vi "4Pi 4Pi Modes - Select Modes.vi"() -> ()   [LabVIEW 2016]
uses:
  4Pi 4Pi Modes - Controls/4Pi 4Pi Modes - Mirror Modes.ctl
  <vilib>/Utility/miscctls.llb/LVPointTypeDef.ctl
  Hardware Configuration/Hardware Configuration Controls/Standard Action.ctl
  4Pi 4Pi Modes - Controls/4Pi 4Pi Modes - Standard Action.ctl
  <userlib>/BMC/BMC.lvlib
panel:
  in  "DM index":string(combo)="0"
  in  "Mirror Modes":T1
  in  "Flags":string="--help"
  in  "Run":bool
  out "error":errorcluster
  out "standard output":string
  out "standard error":string
  in  "Control mode":string(combo)="Single"
  in  "Calling VI Ref":refnum<vi>
  in  "Help":bool
  in  "Quit":bool
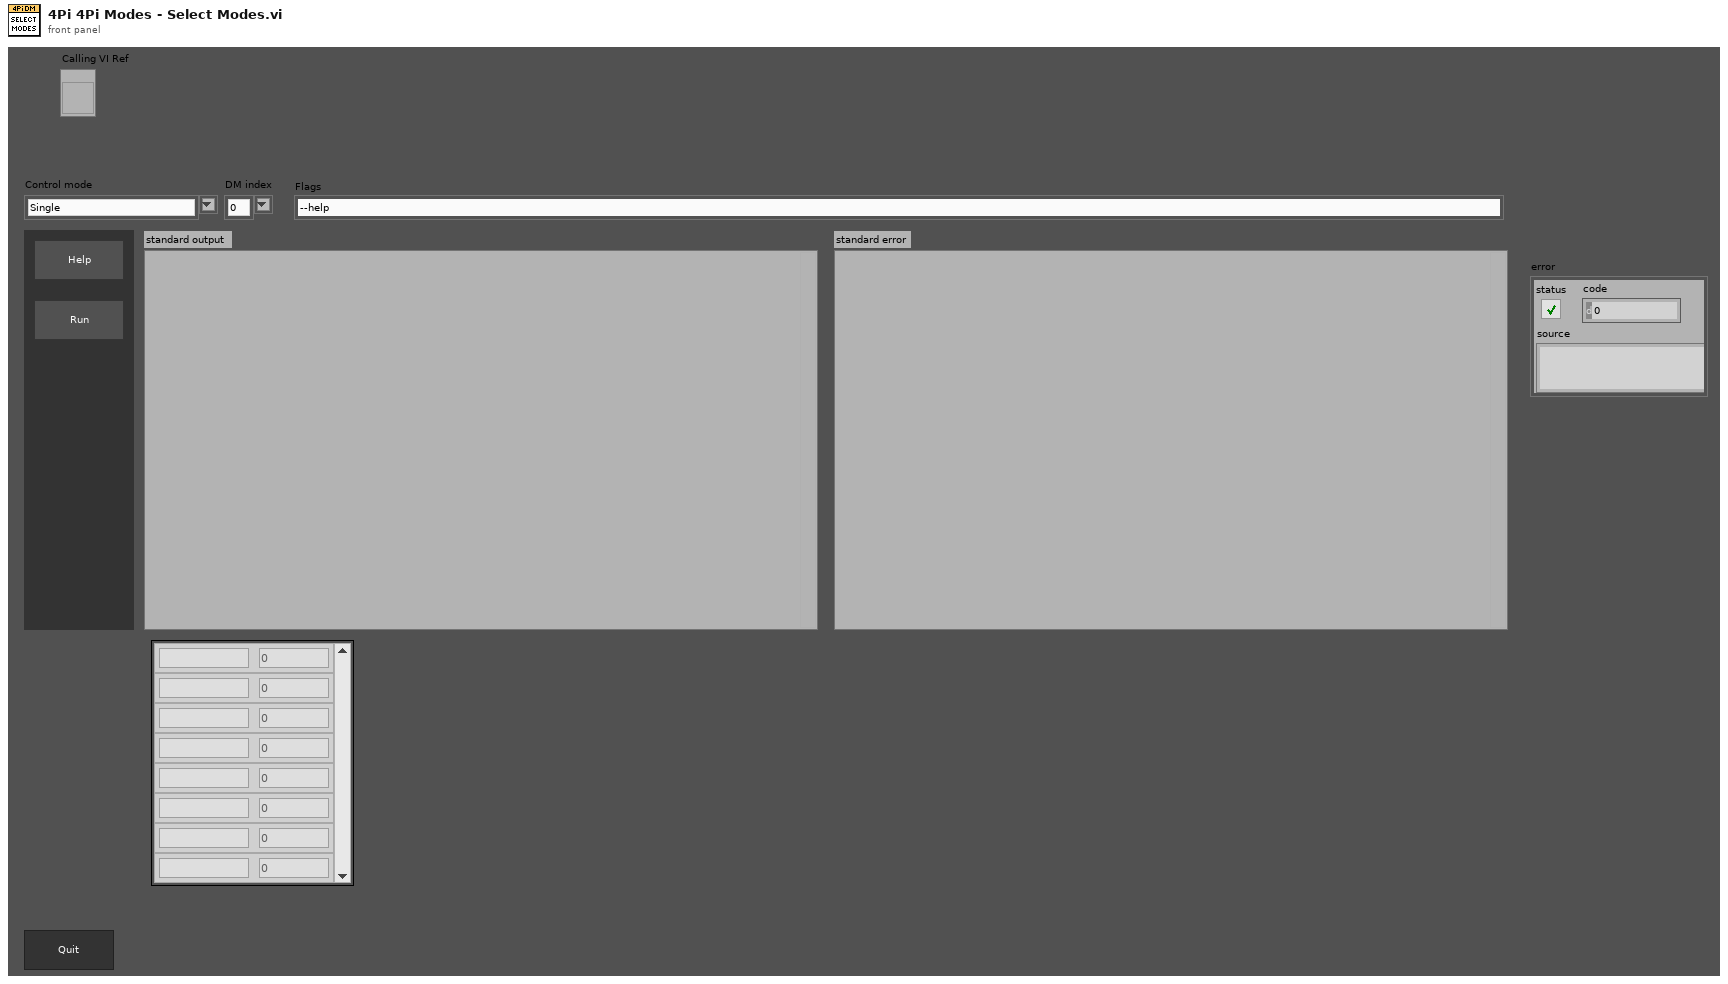
[diagram p1: front panel]
types:
  T1 = typedef "4Pi 4Pi Modes - Mirror Modes.ctl" = cluster{"Mode":string, "Amplitude":dbl}[]
  T2 = enum16{"Always On", "Always Off", "Off While Running"}
  T3 = typedef "LVPointTypeDef.ctl" = cluster{"Horizontal":i16, "Vertical":i16}
  T4 = typedef "Standard Action.ctl" = enum16{"Read", "Write"}
  T5 = typedef "4Pi 4Pi Modes - Standard Action.ctl" = enum16{"Read", "Write"}
  T6 = cluster{"type":i16, "ID":i16, "size":i32, "lutName":u64, "priv":u64}[]
  T7 = typedef "LVRectTypeDef.ctl" = cluster{"Left":i16, "Top":i16, "Right":i16, "Bottom":i16}
  T8 = typedef "LVBoundsTypeDef.ctl" = cluster{"Width":u32, "Height":u32}
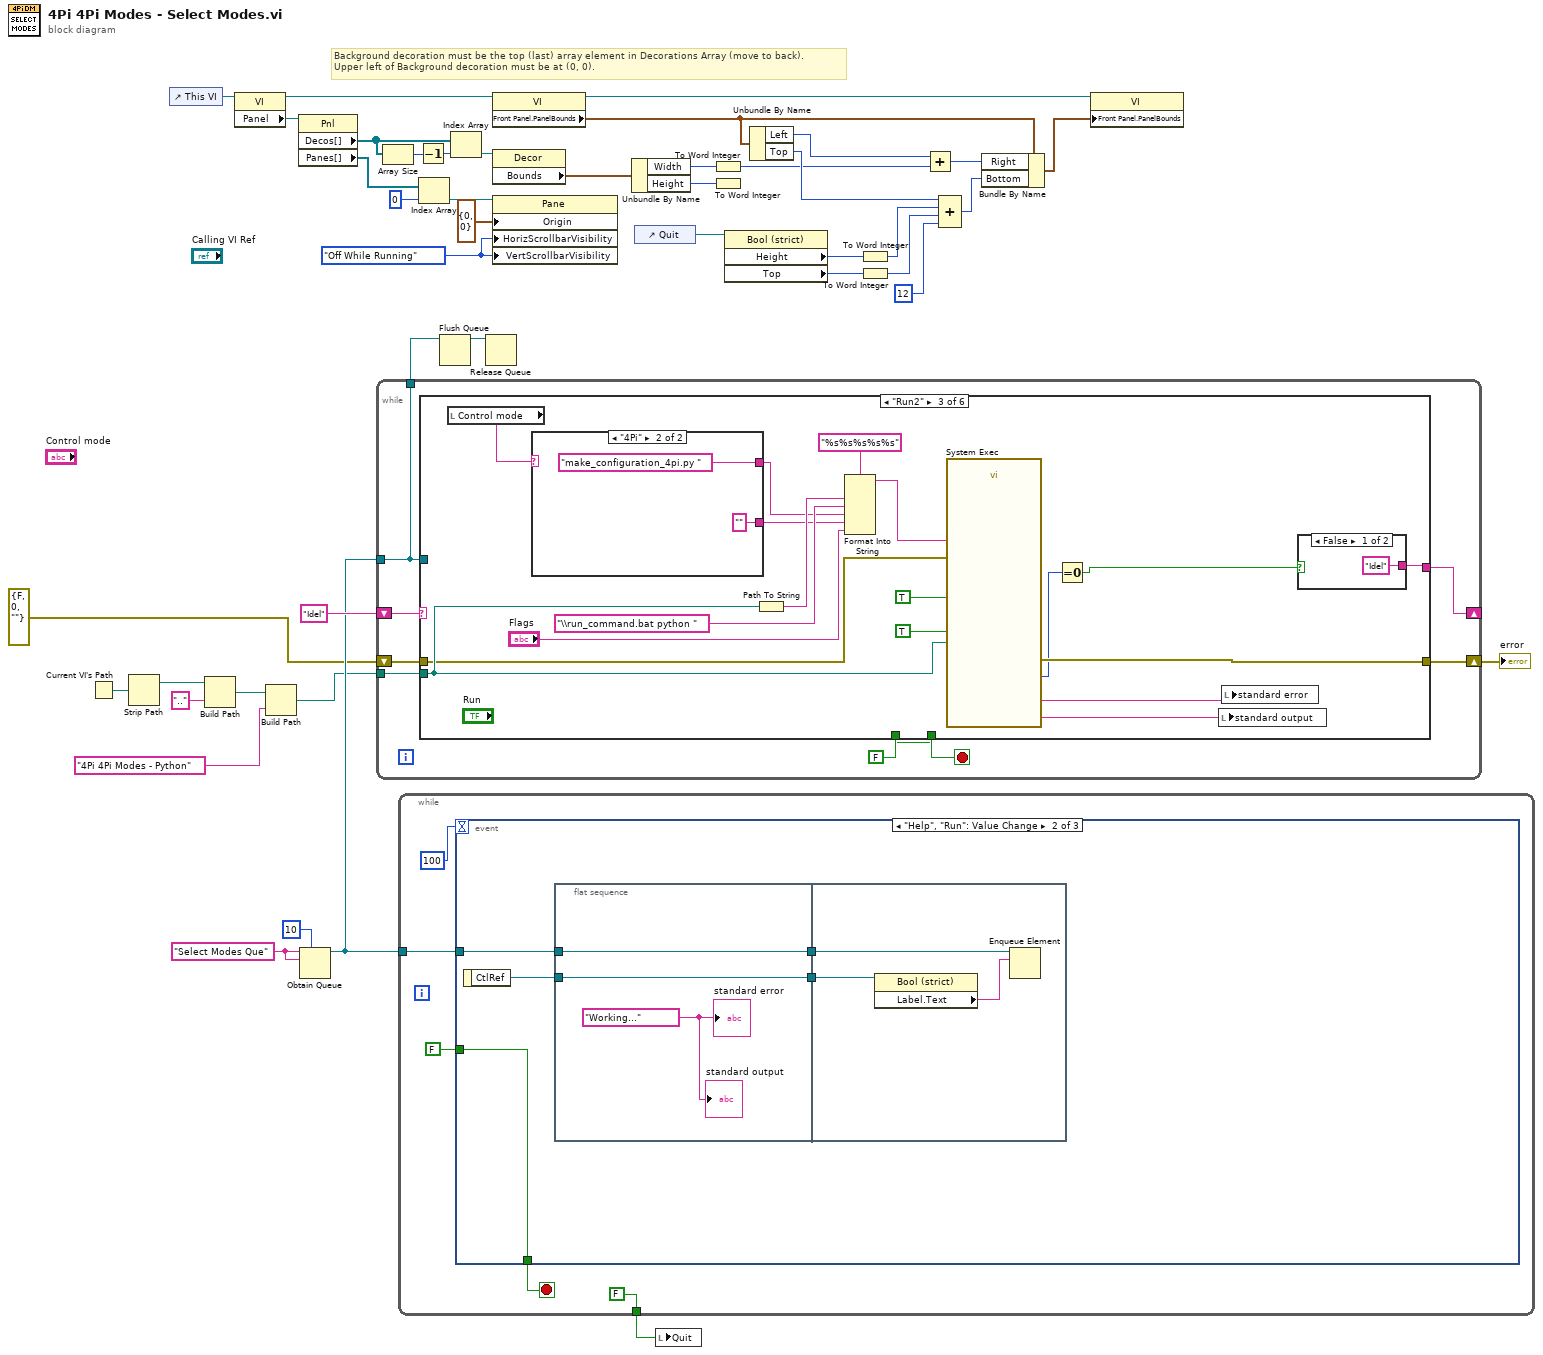
[diagram p0: block diagram]
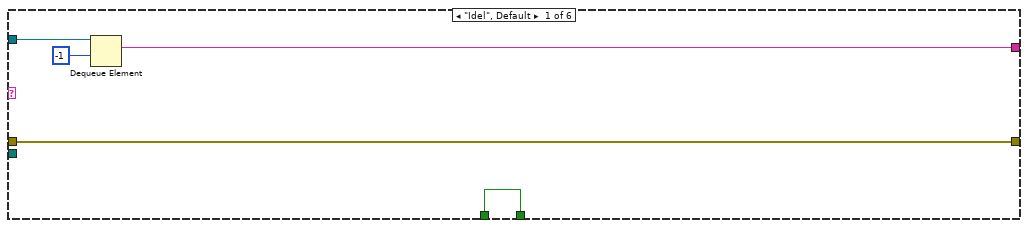
[diagram p2: hidden frame]
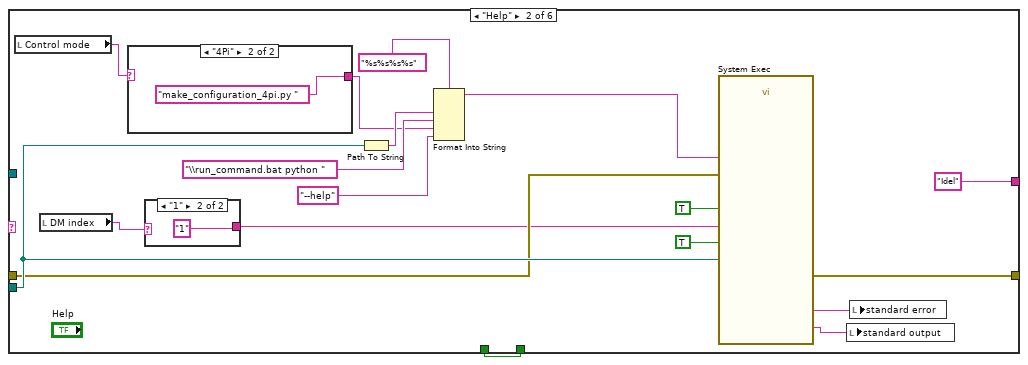
[diagram p3: hidden frame]
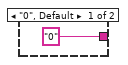
[diagram p4: hidden frame]
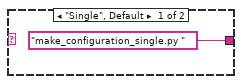
[diagram p5: hidden frame]
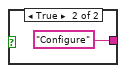
[diagram p6: hidden frame]
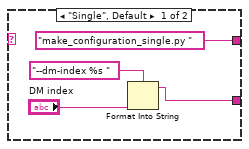
[diagram p7: hidden frame]
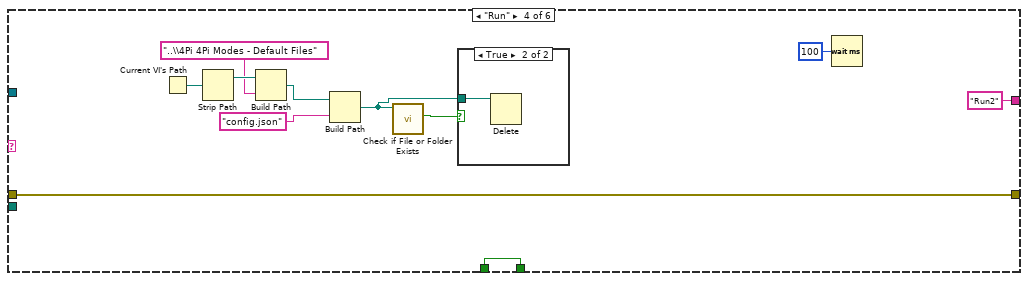
[diagram p8: hidden frame]
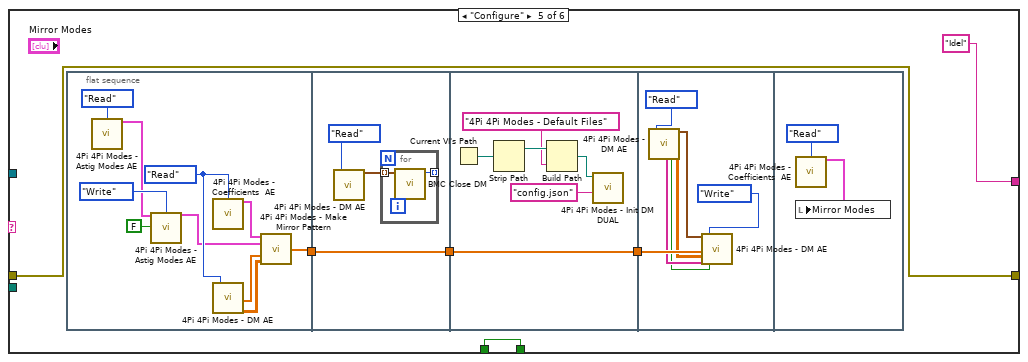
[diagram p10: hidden frame]
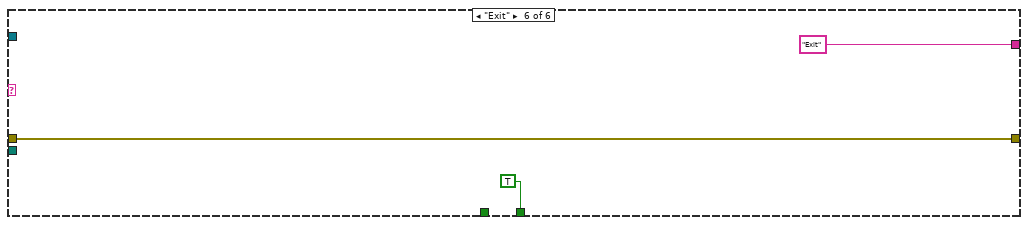
[diagram p11: hidden frame]
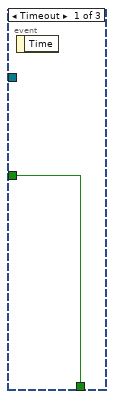
[diagram p12: hidden frame]
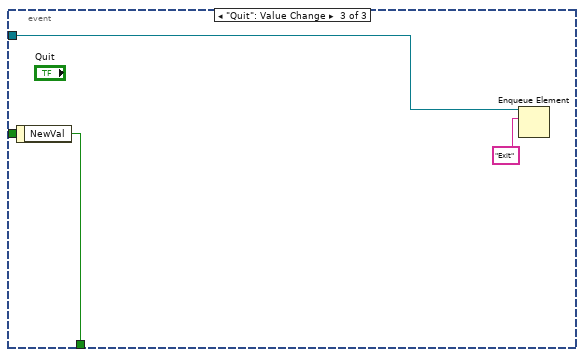
[diagram p13: hidden frame]
diagram:
  w21 = T2."Off While Running" ("Vertical Scrollbar Visibility")
  w44 = "Select Modes Que" ("name (unnamed)")
  # "Background decoration must be the top (last) array element in Decorations Array (move to back).\nUpper left of Background decoration must be at (0, 0)."
  n1 = Current VI's Path() -> (path=w7:path)
  n2 = Strip Path(path=w7) -> (stripped path=w6:path)  [unwired: 1 out]
  n3 = control-ref of="This VI"() -> (w13:refnum<vi>)
  n4 = Build Path(base path=w6, name or relative path="..") -> (appended path=w3:path)
  n5 = property class="VI"(reference=w13) -> (reference out=w22:refnum<vi>, "Panel"=w14:refnum<vi>)  [unwired: 1 in, 1 out]
  n6 = Build Path(base path=w3, name or relative path="4Pi 4Pi Modes - Python") -> (appended path=w4:path)
  n7 = property class="Pnl"(reference=w14) -> ("Decos[]"=w12:refnum<vi>[], "Panes[]"=w18:refnum<vi>[])  [unwired: 1 in, 2 out]
  n8 = Obtain Queue(max queue size (-1, unlimited)=10, name (unnamed)=w44, element data type=w44) -> (queue out=w39:refnum<queue>)  [unwired: 2 in, 2 out]
  n9 = while {
    tunnel: w39 -> [w48]
    shift-right: [w52] -> _
    shift-left: "Idel" ("name (unnamed)") -> [w51]
    tunnel: [w48] -> w42
    tunnel: w4 -> [w47]
    shift-right: [w46] -> w2
    shift-left: errorcluster {"status"=FALSE, "code"=0, "source"=""} ("error out") -> [w45]
    stop <- w50 stop-if-true
    n10 = case shown="\"Run2\"" w51 {
      tunnel: w48 -> [w57 _ _ _ _ _]
      tunnel: [w55 "Idel" ("name (unnamed)") w82 "Run2" ("name (unnamed)") "Idel" ("name (unnamed)") "Exit" ("name (unnamed)")] -> w52
      tunnel: [w54 w74 w98 w110 w119 TRUE] -> w50
      tunnel: FALSE -> [w54 w74 w98 w110 w119 _]
      tunnel: w47 -> [_ w67 w91 _ _ _]
      tunnel: [w53 w60 w86 w111 w120 w155] -> w46
      tunnel: w45 -> [w53 w61 w85 w111 w120 w155]
      frame "Idel", Default {
        n11 = Dequeue Element(queue=w57, timeout in ms (-1)=-1) -> (element=w55:string)  [unwired: 1 in, 3 out]
      }
      frame "Help" {
        n12 = local read "Control mode"() -> (w69:string)
        n13 = local read "DM index"() -> (w59:string)
        n14 = case shown="\"4Pi\"" w69 {
          tunnel: ["make_configuration_single.py " "make_configuration_4pi.py "] -> w63
          frame "Single", Default {
          }
          frame "4Pi" {
          }
        }
        n15 = case shown="\"1\"" w59 {
          tunnel: ["0" ("name or relative path") "1" ("name or relative path")] -> w58
          frame "0", Default {
          }
          frame "1" {
          }
        }
        n16 = Path To String(path=w67) -> (string=w66:string)
        n17 = Format Into String(format string="%s%s%s%s", w66, "\\run_command.bat python " ("name or relative path"), w63, "--help" ("name or relative path")) -> (resulting string=w64:string)  [unwired: 2 in, 1 out]
        n18 = call <vilib>:"System Exec.vi"("run minimized? (F)"=TRUE, "wait until completion? (T)"=TRUE, "error in (no error)"=w61, "working directory"=w67, "standard input"=w58, "command line"=w64) -> ("error out"=w60:errorcluster, "standard error"=w71:string, "standard output"=w70:string)  [unwired: 2 in, 1 out]
        n19 = local write "standard output"(w70) -> ()
        n20 = local write "standard error"(w71) -> ()
      }
      frame "Run2" {
        n21 = local read "Control mode"() -> (w93:string)
        n22 = case shown="\"4Pi\"" w93 {
          tunnel: ["make_configuration_single.py " "make_configuration_4pi.py "] -> w87
          tunnel: [w101 ""] -> w80
          frame "Single", Default {
            n23 = Format Into String(format string="--dm-index %s ", "DM index") -> (resulting string=w101:string)  [unwired: 2 in, 1 out]
          }
          frame "4Pi" {
          }
        }
        n24 = Path To String(path=w91) -> (string=w90:string)
        n25 = Format Into String(format string="%s%s%s%s%s", w90, "\\run_command.bat python " ("name or relative path"), w87, w80, "Flags") -> (resulting string=w88:string)  [unwired: 2 in, 1 out]
        n26 = call <vilib>:"System Exec.vi"("run minimized? (F)"=TRUE, "wait until completion? (T)"=TRUE, "error in (no error)"=w85, "working directory"=w91, "command line"=w88) -> ("error out"=w86:errorcluster, "return code"=w84:i32, "standard error"=w95:string, "standard output"=w94:string)  [unwired: 3 in]
        n27 = Equal To 0?(x=w84) -> (x = 0?=w83:bool)
        n28 = local write "standard output"(w94) -> ()
        n29 = local write "standard error"(w95) -> ()
        n30 = case shown="False" w83 {
          tunnel: ["Idel" ("name (unnamed)") "Configure" ("name (unnamed)")] -> w82
          frame False {
          }
          frame True {
          }
        }
      }
      frame "Run" {
        n31 = Current VI's Path() -> (path=w116:path)
        n32 = Strip Path(path=w116) -> (stripped path=w117:path)  [unwired: 1 out]
        n33 = Build Path(base path=w117, name or relative path="..\\4Pi 4Pi Modes - Default Files") -> (appended path=w114:path)
        n34 = Build Path(base path=w114, name or relative path="config.json") -> (appended path=w107:path)
        n35 = call <vilib>:"Check if File or Folder Exists.vi"("path"=w107) -> ("file or folder exists?"=w108:bool)  [unwired: 8 in, 2 out]
        n36 = case shown="True" w108 {
          tunnel: w107 -> [_ w118]
          frame False {
          }
          frame True {
            n37 = Delete(path (use dialog)=w118) -> ()  [unwired: 4 in, 3 out]
          }
        }
        n38 = Wait (ms)(milliseconds to wait=u32 100) -> ()  [unwired: 1 out]
      }
      frame "Configure" {
        n39 = flat-sequence {
          tunnel: [w125] -> w124
          tunnel: w124 -> [w137]
          tunnel: [w137] -> w123
          tunnel: w123 -> [w140]
          tunnel: [w140] -> w122
          tunnel: w122 -> [w149]
          frame #0 {
            w131 = 4Pi_4Pi_Modes_-_Standard_Action."Read" ("Action")
            n40 = call "4Pi 4Pi Modes - Astig Modes AE.vi"("Action"=Standard_Action."Read") -> ("Coefficients Out"=w126:cluster{"Mode":string, "Amplitude":dbl}[])  [unwired: 13 in, 1 out]
            n41 = call "4Pi 4Pi Modes - Astig Modes AE.vi"("Coefficients In"=w126, "Action"=Standard_Action."Write", "Enabled In"=FALSE) -> ("Coefficients Out"=w129:cluster{"Mode":string, "Amplitude":dbl}[])  [unwired: 11 in, 1 out]
            n42 = call "4Pi 4Pi Modes - Coefficients  AE.vi"("Action"=w131) -> ("Coefficients Out"=w130:cluster{"Mode":string, "Amplitude":dbl}[])  [unwired: 14 in]
            n43 = call "4Pi 4Pi Modes - DM AE.vi"("Action"=w131) -> ("Flats Out"=w128:dbl[], "Control Matrix Out"=w127:dbl[][])  [unwired: 14 in, 3 out]
            n44 = call "4Pi 4Pi Modes - Make Mirror Pattern.vi"("Coefficients"=w130, "Astig Coeffs"=w129, "Flats"=w128, "Control Matrix"=w127) -> ("Pixel Value U (-1 to 1)"=w125:dbl[])  [unwired: 10 in, 1 out]
          }
          frame #1 {
            n45 = call "4Pi 4Pi Modes - DM AE.vi"("Action"=4Pi_4Pi_Modes_-_Standard_Action."Read") -> ("DM Handles Out"=w135:T6)  [unwired: 14 in, 4 out]
            n46 = for {
              tunnel: w135 -> [w139] mode=indexing
              tunnel: [w138] -> _ mode=indexing
              n47 = call <userlib>:"BMC Close DM.vi"("dmHandle"=w139) -> ("function return"=w138:i32)  [unwired: 9 in, 1 out]
            }
          }
          frame #2 {
            n48 = Current VI's Path() -> (path=w142:path)
            n49 = Strip Path(path=w142) -> (stripped path=w143:path)  [unwired: 1 out]
            n50 = Build Path(base path=w143, name or relative path="4Pi 4Pi Modes - Default Files") -> (appended path=w145:path)
            n51 = call "4Pi 4Pi Modes - Init DM DUAL.vi"("Config File"="config.json" ("name or relative path"), "Base File Path"=w145) -> ()  [unwired: 8 in, 2 out]
          }
          frame #3 {
            n52 = call "4Pi 4Pi Modes - DM AE.vi"("Action"=4Pi_4Pi_Modes_-_Standard_Action."Read") -> ("Serials Out"=w147:string[], "No hardware Out"=w146:bool, "DM Handles Out"=w150:T6, "Control Matrix Out"=w148:dbl[][])  [unwired: 14 in, 1 out]
            n53 = call "4Pi 4Pi Modes - DM AE.vi"("DM Handles"=w150, "Flats"=w149, "Control Matrix"=w148, "Serials"=w147, "Action"=4Pi_4Pi_Modes_-_Standard_Action."Write", "No hardware"=w146) -> ()  [unwired: 9 in, 5 out]
          }
          frame #4 {
            n54 = call "4Pi 4Pi Modes - Coefficients  AE.vi"("Action"=4Pi_4Pi_Modes_-_Standard_Action."Read") -> ("Coefficients Out"=w153:cluster{"Mode":string, "Amplitude":dbl}[])  [unwired: 14 in]
            n55 = local write "Mirror Modes"(w153) -> ()
          }
        }
      }
      frame "Exit" {
      }
    }
  }
  "error" <- w2
  n56 = Array Size(array=w12) -> (size(s)=w10:i32)
  n57 = while {
    tunnel: w39 -> [w159]
    tunnel: [FALSE] -> w9
    stop <- w162 stop-if-true
    n58 = event shown="[1] \"Help\", \"Run\": Value Change" {
      selector: _ -> [_ _ _]
      dyn-events: _ -> [_ _ _]
      timeout: 100 -> [_ _ _]
      tunnel: [w163 w168 w177] -> w162
      tunnel: FALSE -> [w163 w168 _]
      tunnel: w159 -> [_ w167 w175]
      event Timeout {
        n59 = event-data() -> ()  [unwired: 1 in, 1 out]
      }
      event "Help", "Run": Value Change {
        n60 = event-data() -> ("CtlRef"=w166:refnum<vi>)  [unwired: 1 in]
        n61 = flat-sequence {
          tunnel: w166 -> [w170]
          tunnel: w167 -> [w171]
          tunnel: [w171] -> w165
          tunnel: [w170] -> w164
          tunnel: w165 -> [w174]
          tunnel: w164 -> [w173]
          frame #0 {
            w169 = "Working..." ("standard error")
            "standard error" <- w169
            "standard output" <- w169
          }
          frame #1 {
            n62 = property class="Bool (strict)"(reference=w173) -> ("Label.Text"=w172:string)  [unwired: 1 in, 2 out]
            n63 = Enqueue Element(queue=w174, element=w172) -> ()  [unwired: 2 in, 3 out]
          }
        }
      }
      event "Quit": Value Change {
        n64 = event-data() -> ("NewVal"=w177:bool)  [unwired: 1 in]
        n65 = Enqueue Element(queue=w175, element="Exit") -> ()  [unwired: 2 in, 3 out]
      }
    }
  }
  n66 = Decrement(x=w10) -> (x-1=w11:i32)
  n67 = Index Array(array=w18, index=0) -> (element=w17:refnum<vi>)
  n68 = Flush Queue(queue=w42) -> (queue out=w41:refnum<queue>)  [unwired: 1 in, 2 out]
  n69 = Index Array(array=w12, index=w11) -> (element=w20:refnum<vi>)
  n70 = Release Queue(queue=w41) -> ()  [unwired: 2 in, 3 out]
  n71 = property class="VI"(reference=w22) -> (reference out=w24:refnum<vi>, "Front Panel.PanelBounds"=w25:T7)  [unwired: 1 in, 1 out]
  n72 = property class="Decor"(reference=w20) -> ("Bounds"=w23:T8)  [unwired: 1 in, 2 out]
  n73 = property class="Pane"(reference=w17, "Origin"=T3 {"Horizontal"=0, "Vertical"=0}, "HorizScrollbarVisibility"=w21, "VertScrollbarVisibility"=w21) -> ()  [unwired: 1 in, 2 out]
  n74 = Unbundle By Name(w23) -> ("Width"=w28:u32, "Height"=w31:u32)
  n75 = control-ref of="Quit"() -> (w15:refnum<vi>)
  n76 = local write "Quit"(w9) -> ()
  n77 = To Word Integer(number=w28) -> (16bit integer=w30:i16)
  n78 = To Word Integer(number=w31) -> ()  [unwired: 1 out]
  n79 = property class="Bool (strict)"(reference=w15) -> ("Height"=w33:u32, "Top"=w34:i32)  [unwired: 1 in, 2 out]
  n80 = Unbundle By Name(w25) -> ("Left"=w27:i16, "Top"=w38:i16)
  n81 = To Word Integer(number=w33) -> (16bit integer=w36:i16)
  n82 = To Word Integer(number=w34) -> (16bit integer=w37:i16)
  n83 = Add(x=w27, y=w30) -> (x+y=w29:i16)
  n84 = Compound Arithmetic op=ADD(w38, w36, w37, i16 12 ("y")) -> (w32:i16)
  n85 = Bundle By Name(cluster=w25, "Right"=w29, "Bottom"=w32) -> (w26:T7)
  n86 = property class="VI"(reference=w24, "Front Panel.PanelBounds"=w26) -> ()  [unwired: 1 in, 2 out]
